vi "MISC Search String Array.vi"(9 "Case Sensitive (T)":bool=TRUE, 10 "String":string, 11 "String Array":string[](array[string])) -> (0 "All Indeces":i32[](array[numeric]), 1 "All Elements":string[](array[string]), 2 "First Index":i32, 3 "First Element":string, 5 "Last Element":string)   [LabVIEW 2012]
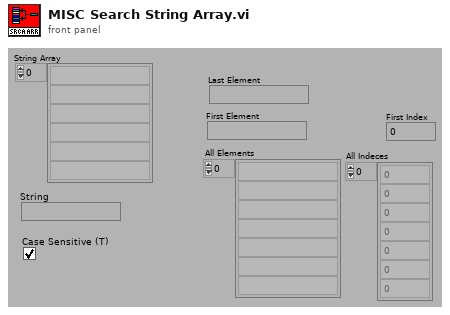
[diagram p1: front panel]
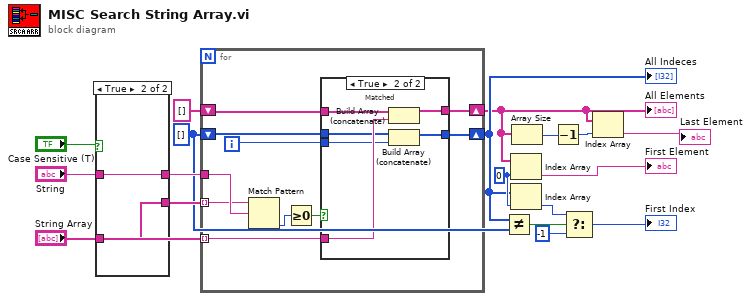
[diagram p0: block diagram]
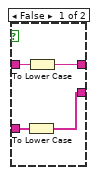
[diagram p2: hidden frame]
diagram:
  w16 = 0
  w10 = i32[] []
  n1 = case shown="True" "Case Sensitive (T)" {
    tunnel: [w20 w24] -> w13
    tunnel: "String" -> [w22 w24]
    tunnel: "String Array" -> [w21 w23]
    tunnel: [w19 w23] -> w12
    frame False {
      n2 = To Lower Case(string=w21) -> (all lower case string=w19:string[])
      n3 = To Lower Case(string=w22) -> (all lower case string=w20:string)
    }
    frame True {
    }
  }
  n4 = for {
    tunnel: "String Array" -> [w32] mode=indexing
    tunnel: w13 -> [w34]
    shift-right: [w31] -> w2
    shift-left: string[] [] -> [w30]
    shift-right: [w29] -> w9
    shift-left: w10 -> [w28]
    tunnel: w12 -> [w25] mode=indexing
    i -> [w26]
    n5 = Match Pattern(string=w25, regular expression=w34) -> (offset past match=w27:i32)  [unwired: 4 out]
    n6 = Greater Or Equal To 0?(x=w27) -> (x >= 0?=w33:bool)
    n7 = case shown="True" w33 {
      tunnel: w32 -> [_ w42]
      tunnel: [w36 w41] -> w31
      tunnel: w30 -> [w36 w40]
      tunnel: w26 -> [_ w39]
      tunnel: [w35 w38] -> w29
      tunnel: w28 -> [w35 w37]
      frame False {
        # "Not Matched"
      }
      frame True {
        # "Matched"
        n8 = Build Array (concatenate)(w40, w42) -> (w41:string[])
        n9 = Build Array (concatenate)(w37, w39) -> (w38:i32[])
      }
    }
  }
  "All Indeces" <- w9
  "All Elements" <- w2
  n10 = Not Equal?(x=w9, y=w10) -> (x != y?=w8:bool)
  n11 = Index Array(array=w2, index=w16) -> (element=→"First Element":string)
  n12 = Index Array(array=w9, index=w16) -> (element=w7:i32)
  n13 = Array Size(array=w2) -> (size(s)=w4:i32)
  n14 = Decrement(x=w4) -> (x-1=w3:i32)
  n15 = Select(t=w7, s=w8, f=-1) -> (s? t:f=→"First Index":i32)
  n16 = Index Array(array=w2, index=w3) -> (element=→"Last Element":string)
